vi "双随机相减温度.vi"() -> ()   [LabVIEW 2018]
panel:
  out "温度计":dbl(slide) scale=-100.0..100.0
  out "波形图表":dbl(graph)
  in  "停止":bool
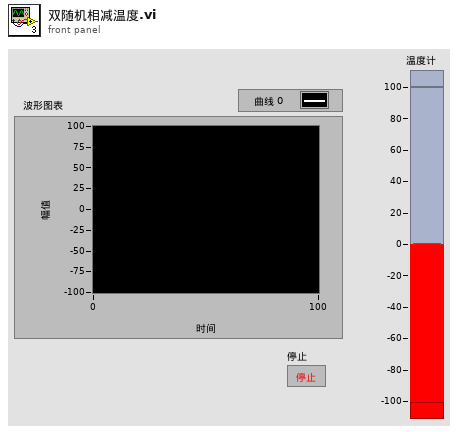
[diagram p1: front panel]
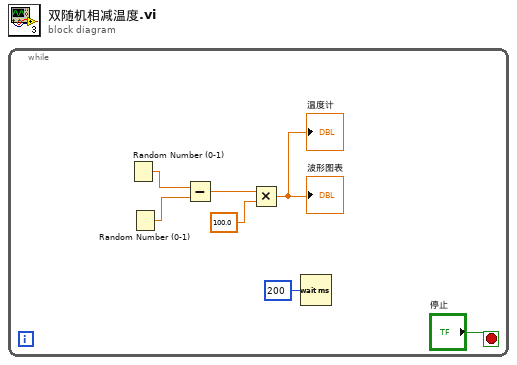
[diagram p0: block diagram]
diagram:
  n1 = while {
    stop <- "停止" stop-if-true
    n2 = Random Number (0-1)() -> (number: 0 to 1=w7:dbl)
    n3 = Random Number (0-1)() -> (number: 0 to 1=w6:dbl)
    n4 = Subtract(x=w7, y=w6) -> (x-y=w5:dbl)
    n5 = Multiply(x=w5, y=100.0 ("x")) -> (x*y=→"波形图表" →"温度计":dbl)
    n6 = Wait (ms)(milliseconds to wait=u32 200 ("等待时间（毫秒）")) -> ()  [unwired: 1 out]
  }
